vi "FlatToRichpumploop_Sensors.vi"(5 "OutputClusterType":T1, 11 "InputCluster":T2) -> (3 "OutputCluster":T1)   [LabVIEW 2024, in "pumploop_client.lvlib"]
uses:
  pumploop_client.lvlib
  pumploop_Sensors_Flat.ctl
  pumploop_Sensors.ctl
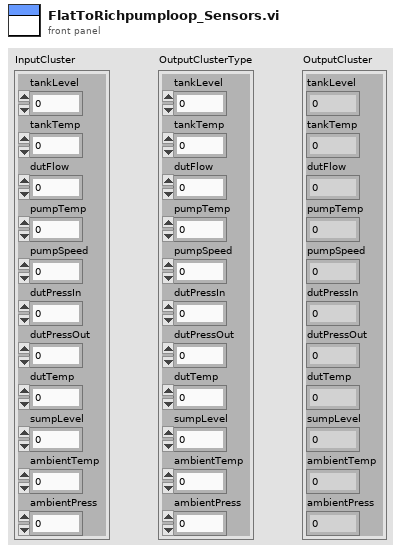
[diagram p1: front panel]
types:
  T1 = typedef "pumploop_client.lvlib/pumploop_Sensors.ctl" = cluster{"tankLevel":sgl, "tankTemp":sgl, "dutFlow":sgl, "pumpTemp":sgl, "pumpSpeed":sgl, "dutPressIn":sgl, "dutPressOut":sgl, "dutTemp":sgl, "sumpLevel":sgl, "ambientTemp":sgl, "ambientPress":sgl}
  T2 = typedef "pumploop_client.lvlib/pumploop_Sensors_Flat.ctl" = cluster{"tankLevel":sgl, "tankTemp":sgl, "dutFlow":sgl, "pumpTemp":sgl, "pumpSpeed":sgl, "dutPressIn":sgl, "dutPressOut":sgl, "dutTemp":sgl, "sumpLevel":sgl, "ambientTemp":sgl, "ambientPress":sgl}
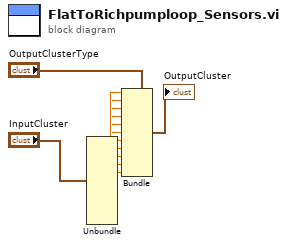
[diagram p0: block diagram]
diagram:
  n1 = Unbundle "Unbundle"("InputCluster") -> ("tankLevel"=w11:sgl, "tankTemp"=w10:sgl, "dutFlow"=w9:sgl, "pumpTemp"=w8:sgl, "pumpSpeed"=w7:sgl, "dutPressIn"=w6:sgl, "dutPressOut"=w5:sgl, "dutTemp"=w4:sgl, "sumpLevel"=w3:sgl, "ambientTemp"=w2:sgl, "ambientPress"=w1:sgl)
  n2 = Bundle "Bundle"(cluster="OutputClusterType", "tankLevel"=w11, "tankTemp"=w10, "dutFlow"=w9, "pumpTemp"=w8, "pumpSpeed"=w7, "dutPressIn"=w6, "dutPressOut"=w5, "dutTemp"=w4, "sumpLevel"=w3, "ambientTemp"=w2, "ambientPress"=w1) -> (→"OutputCluster":T1)
